vi "FlatToRichrouteguide_response.vi"(5 "OutputClusterType":T1, 11 "InputCluster":T3) -> (3 "OutputCluster":T1)   [LabVIEW 2019, in "Generated_server.lvlib"]
uses:
  Generated_server.lvlib
  routeguide_response_Flat.ctl
  routeguide_Color.ctl
  routeguide_response.ctl
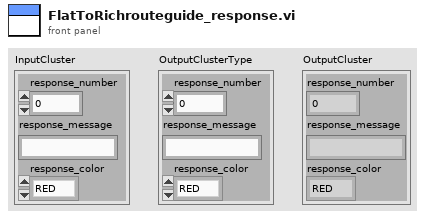
[diagram p1: front panel]
types:
  T1 = typedef "Generated_server.lvlib/routeguide_response.ctl" = cluster{"response_number":i32, "response_message":string, "response_color":T2}
  T2 = typedef "Generated_server.lvlib/routeguide_Color.ctl" = enum32{"RED", "GREEN", "BLUE"}
  T3 = typedef "Generated_server.lvlib/routeguide_response_Flat.ctl" = cluster{"response_number":i32, "response_message":string, "response_color":T2}
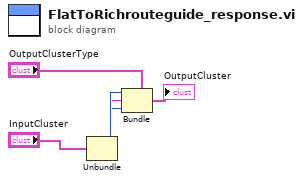
[diagram p0: block diagram]
diagram:
  n1 = Unbundle "Unbundle"("InputCluster") -> ("response_number"=w3:i32, "response_message"=w2:string, "response_color"=w1:T2)
  n2 = Bundle "Bundle"(cluster="OutputClusterType", "response_number"=w3, "response_message"=w2, "response_color"=w1) -> (→"OutputCluster":T1)
